vi "createImg.vi"(7 "label":string, 8 "error in (no error)":errorcluster, 9 "path":string, 10 "seg ref":refnum<k20>, 11 "DOM document":refnum<k20>) -> (0 "error out":errorcluster, 2 "dup seg ref":refnum<k20>, 3 "dup DOM document":refnum<k20>)   [LabVIEW 2013]
uses:
  <vilib>/xml/Close Reference(Node).vi
  <resource>/objmgr/DOMUserDefRef.rc
  <vilib>/xml/NI_XML.lvlib
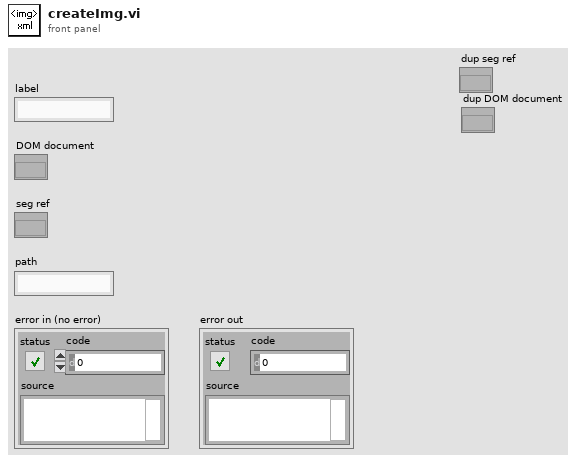
[diagram p1: front panel]
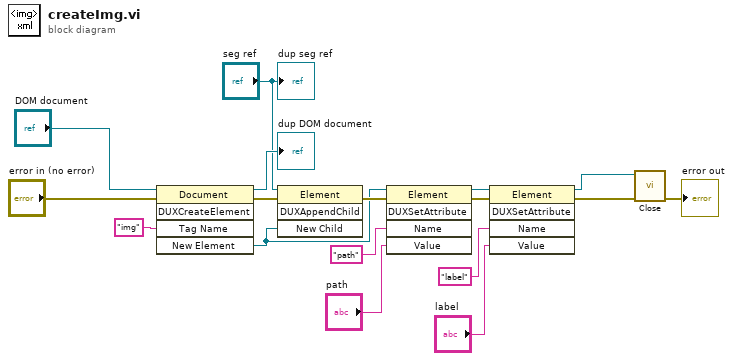
[diagram p0: block diagram]
diagram:
  n1 = invoke class="Document" method="DUXCreateElement"(reference="DOM document", error in="error in (no error)", "Tag Name"="img") -> (reference out=→"dup DOM document":refnum<k20>, error out=w8:errorcluster, "New Element"=w4:refnum<k20>)  [unwired: 2 in, 2 out]
  n2 = invoke class="Element" method="DUXAppendChild"(reference="seg ref", error in=w8, "New Child"=w4) -> (error out=w10:errorcluster)  [unwired: 1 in, 3 out]
  n3 = invoke class="Element" method="DUXSetAttribute"(reference=w4, error in=w10, "Name"="path", "Value"="path") -> (reference out=w13:refnum<k20>, error out=w14:errorcluster)  [unwired: 1 in, 3 out]
  n4 = invoke class="Element" method="DUXSetAttribute"(reference=w13, error in=w14, "Name"="label", "Value"="label") -> (reference out=w1:refnum<k20>, error out=w3:errorcluster)  [unwired: 1 in, 3 out]
  n5 = call-poly <vilib>:"Close.vi"("error in (no error)"=w3, "node"=w1) -> ("error out"=→"error out":errorcluster)  [unwired: 7 out]
  "dup seg ref" <- "seg ref"
